vi "InertialControl.vi"() -> ()   [LabVIEW 2019]
doc: "high-level user control for inertial control"
uses:
  D:/Victor Sun/optical trap control/Kinesis/Thorlabs.MotionControl.Controls.dll
  Kinesis/Thorlabs.MotionControl.Controls.dll
  D:/Victor Sun/optical trap control/Kinesis/Thorlabs.MotionControl.KCube.InertialMotorCLI.dll
  Kinesis/Thorlabs.MotionControl.KCube.InertialMotorCLI.dll
panel:
  out "current state":string
  in  "stop data write loop":bool
  in  "start/stop write":bool
  in  "init file":bool
  in  "Folder path save":path
  in  "filename save":string="D:\\Victor Sun\\optical trap control\\output_test\\testposition"
  in  "decrease/reverse":bool
  in  "JogStepRev in":i32=250
  in  "JogStepFwd out":i32=500
  in  "position":i32
  in  "move to?":bool
  in  "increase/forward":bool
  out "JogStepRev out":i32
  out "JogStepFwd out":i32
  out "JogRate":i32
  out "JogAcceleration":i32
  out "JogMode":i32(ring)=1 items=["Continuous"=1, "Step"=2]
  out "StepRate":i32
  out "StepAcceleration":i32
  out "MaxVoltage":i32
  in  "stop motors":bool
  out "GetPosition":i32
  in  "Stop Button":bool
  in  "SerialNumber 2":string="97000019"
  in  "KCubeInertialMotorControl":refnum<k24>(container)
  # "Low-level parameters (which one of these to include)"
  # "Relative Position Control"
  # "Data Acquisition Settings"
  # "Absolute Position Control"
  # "Goto"
  # "Jog"
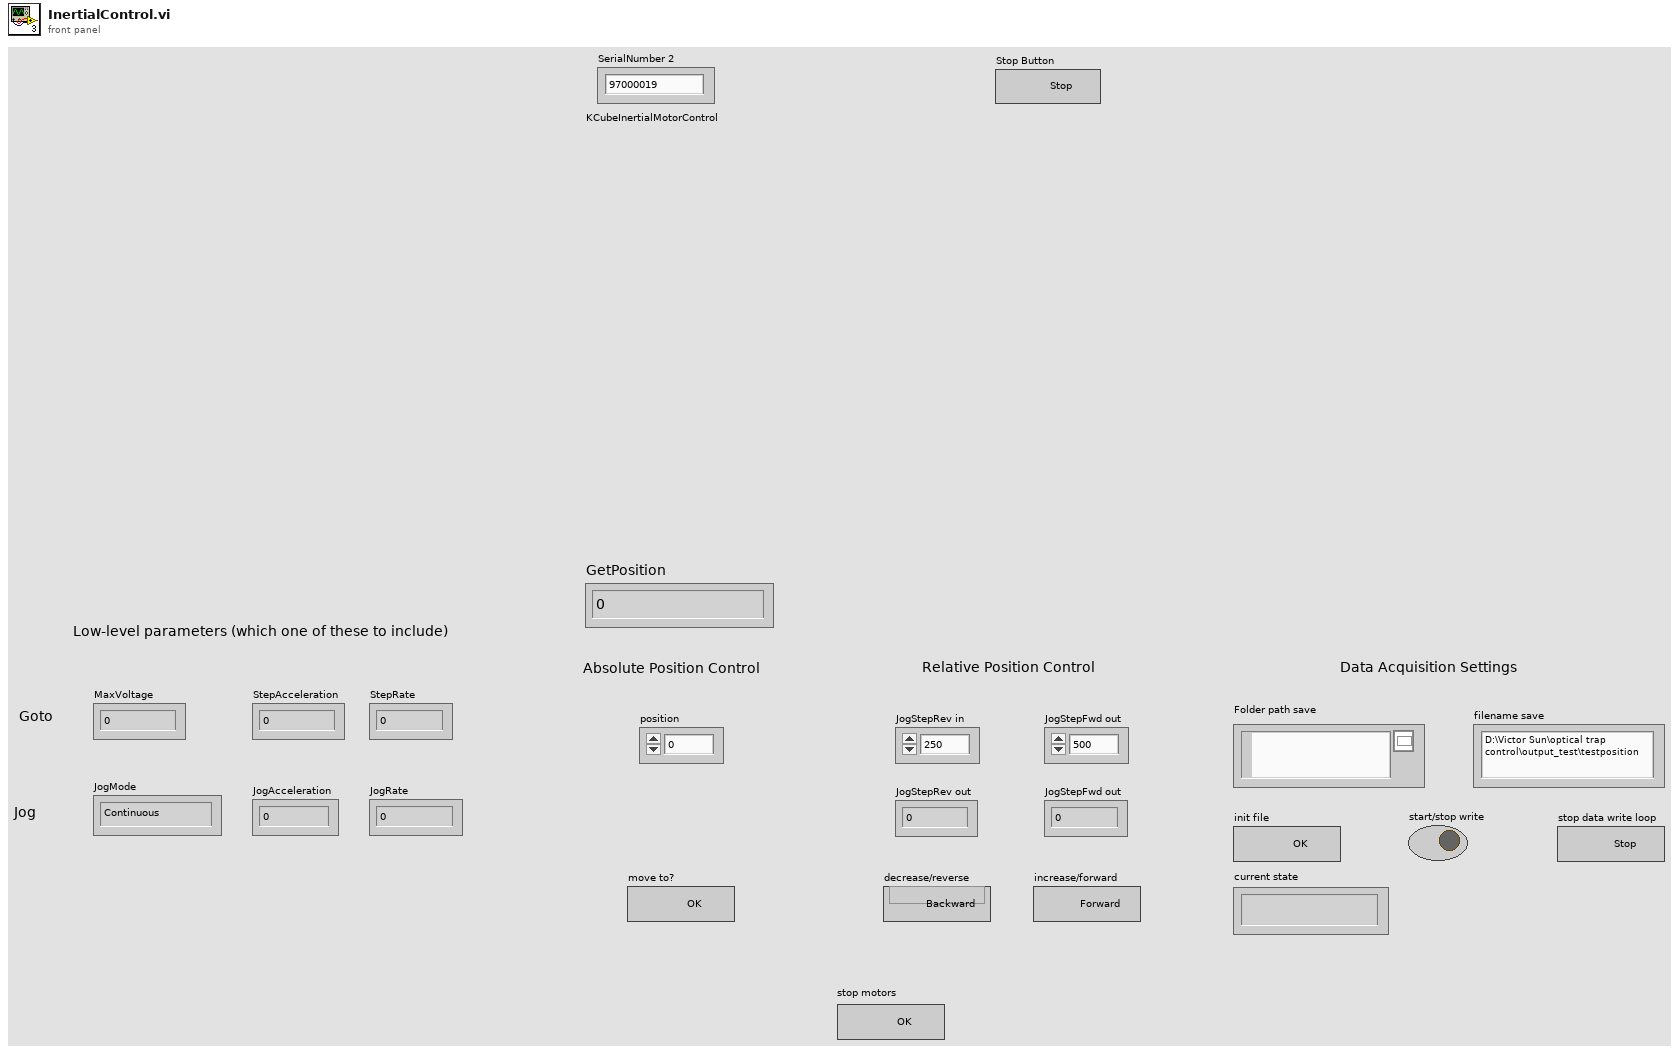
[diagram p1: front panel]
types:
  T1 = enum16{"waiting for init", "init", "waiting for write", "write", "stop"}
  T2 = cluster{"StepRate":i32, "StepAcceleration":i32, "MaxVoltage":i32}
  T3 = enum16{"waiting for init", "init", "waiting for write", "write", "stop", ""}
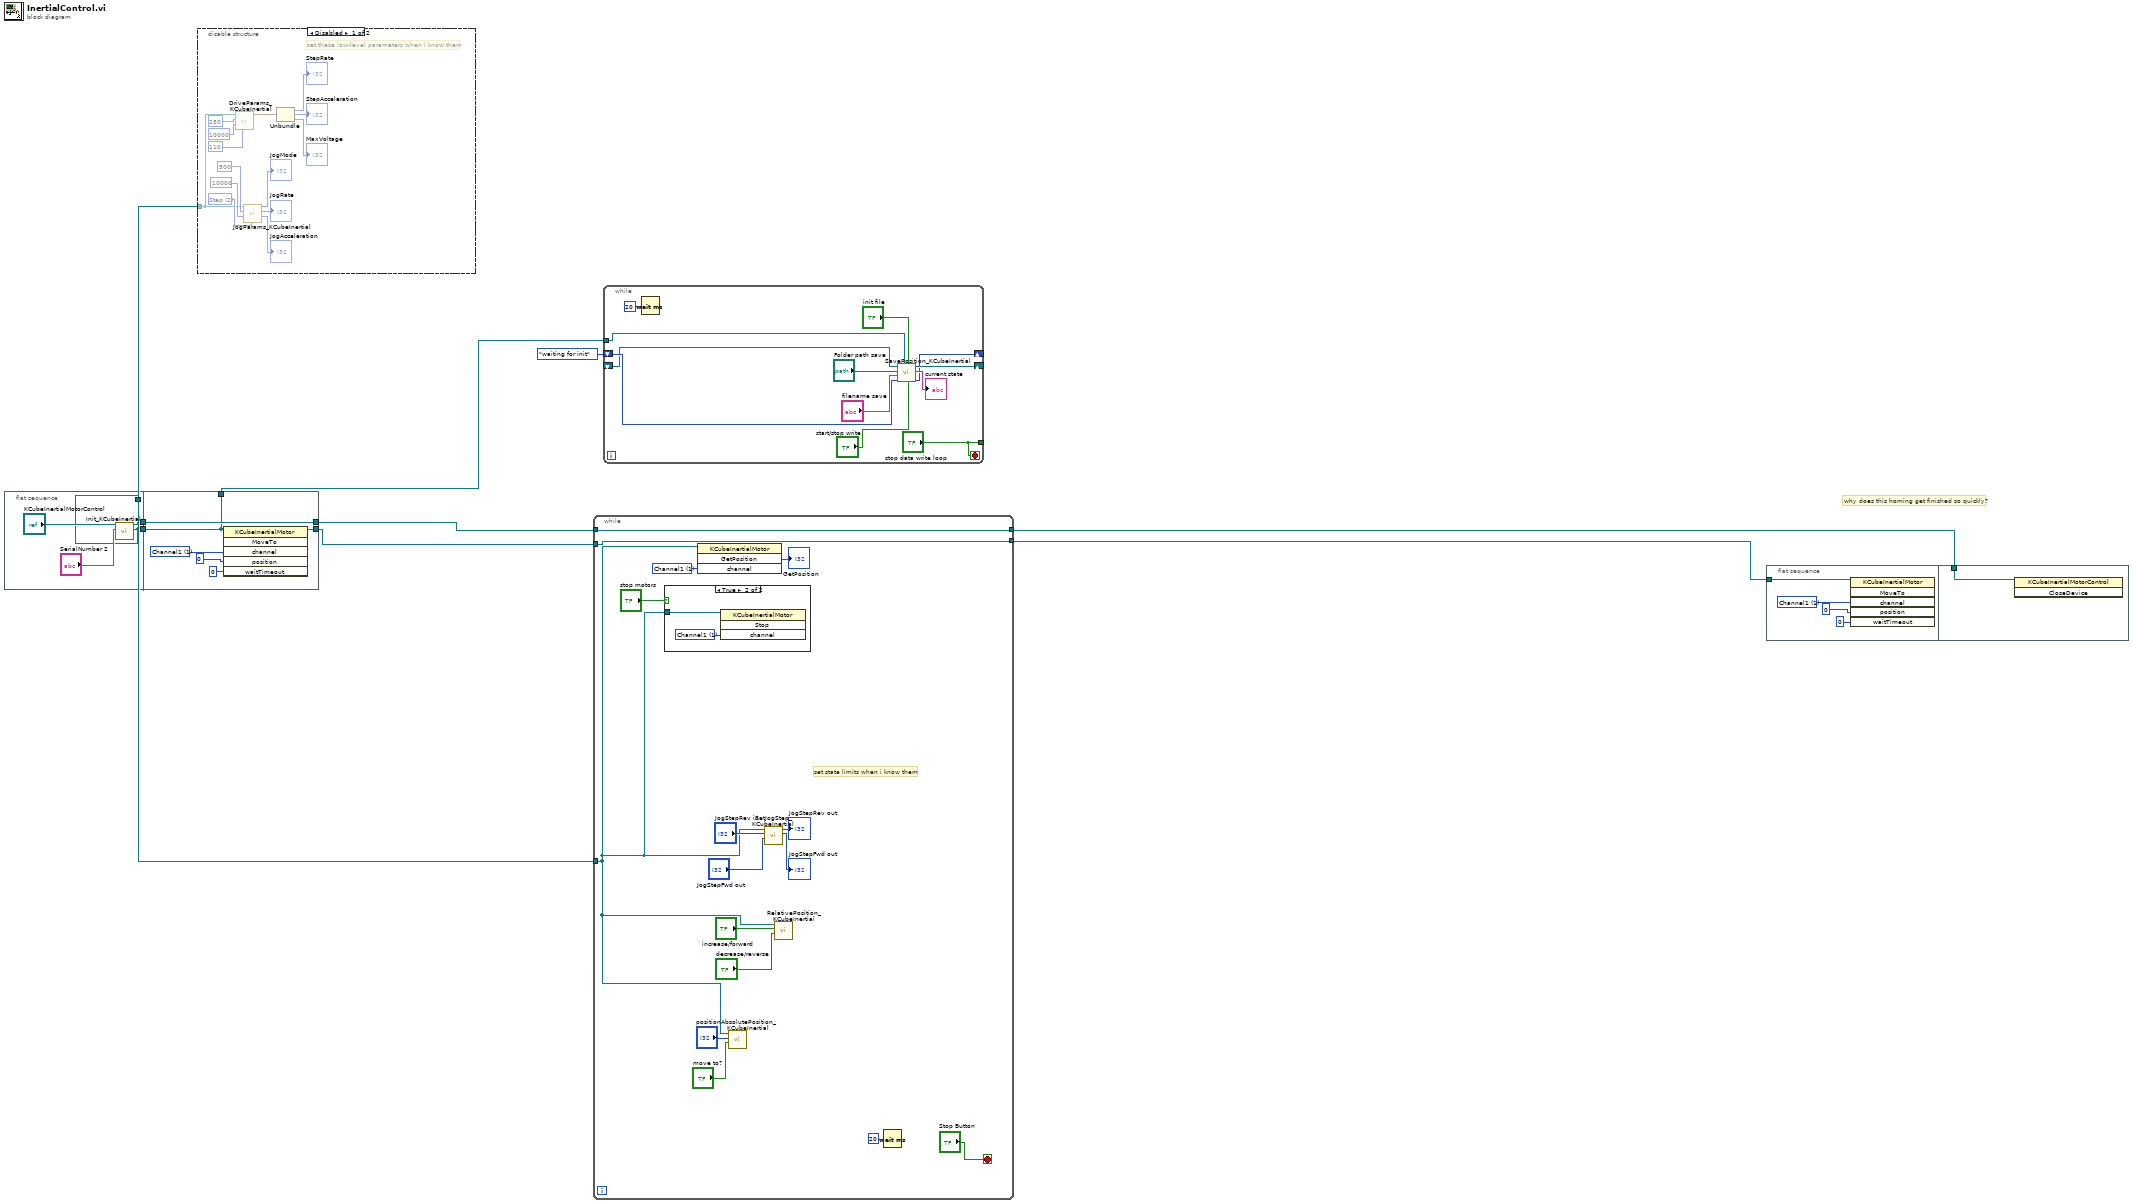
[diagram p0: block diagram]
diagram:
  # "why does this homing get finished so quickly?"
  n1 = flat-sequence {
    tunnel: [w10] -> w8
    tunnel: [w12] -> w6
    tunnel: [w10] -> w5
    tunnel: [w19] -> w9
    tunnel: w6 -> [w19]
    tunnel: w5 -> [w14]
    tunnel: [w15] -> w4
    tunnel: [w14] -> w1
    frame #0 {
      n2 = call "Init_KCubeInertial.vi"("SerialNumber in"="SerialNumber 2", ".NET Refnum in"="KCubeInertialMotorControl") -> ("Device"=w10:refnum<k24>, ".NET Refnum out"=w12:refnum<k24>)  [unwired: 7 in, 1 out]
    }
    frame #1 {
      w18 = 1 items=["Channel1"=1, "Channel2"=2, "Channel3"=3, "Channel4"=4] ("channel")
      n3 = invoke class="KCubeInertialMotor" method="MoveTo"(reference=w14, "channel"=w18, "position"=0, "waitTimeout"=0) -> (reference out=w15:refnum<k24>)  [unwired: 2 in, 5 out]
    }
  }
  n4 = disable-structure shown="Disabled" {
    disable-tunnel: w8 -> [w20 _]
    frame Disabled {
      w23 = 2 items=["Continuous"=1, "Step"=2] ("JogMode")
      # "set these low-level parameters when i know them"
      n5 = call "DriveParams_KCubeInertial.vi"("MaxVoltage"=110, "StepAcceleration"=10000, "StepRate"=250, ".NET Refnum in"=w20) -> ("Cluster"=w30:T2)  [unwired: 7 in]
      n6 = call "JogParams_KCubeInertial.vi"("JogMode in"=w23, "JogAcceleration in"=10000 ("JogAcceleration"), "JogRate in"=500 ("JogRate"), ".NET Refnum in"=w20) -> ("JogAcceleration out"=→"JogAcceleration":i32, "JogRate out"=→"JogRate":i32, "JogMode out"=→"JogMode":i32)  [unwired: 5 in]
      n7 = Unbundle(w30) -> ("StepRate"=→"StepRate":i32, "StepAcceleration"=→"StepAcceleration":i32, "MaxVoltage"=→"MaxVoltage":i32)
    }
    frame Enabled {
    }
  }
  n8 = while {
    tunnel: w9 -> [w48]
    tunnel: [w48] -> w7
    tunnel: w8 -> [w35]
    tunnel: w4 -> [w34]
    tunnel: [w34] -> w3
    stop <- "Stop Button" stop-if-true
    w46 = 1 items=["Channel1"=1, "Channel2"=2, "Channel3"=3, "Channel4"=4] ("channel")
    # "set state limits when i know them"
    n9 = case shown="True" "stop motors" {
      tunnel: w35 -> [_ w50]
      frame False {
      }
      frame True {
        w51 = 1 items=["Channel1"=1, "Channel2"=2, "Channel3"=3, "Channel4"=4] ("channel")
        n10 = invoke class="KCubeInertialMotor" method="Stop"(reference=w50, "channel"=w51) -> ()  [unwired: 2 in, 4 out]
      }
    }
    n11 = invoke class="KCubeInertialMotor" method="GetPosition"(reference=w35, "channel"=w46) -> ("GetPosition"=→"GetPosition":i32)  [unwired: 2 in, 3 out]
    n12 = call "AbsolutePosition_KCubeInertial.vi"("go to?"="move to?", "set absolute position"="position", ".NET Refnum in"=w35) -> ()  [unwired: 9 in]
    n13 = call "SetJogStep_KCubeInertial.vi"("JogStepFwd in"="JogStepFwd out", "JogStepRev in"="JogStepRev in", ".NET Refnum in"=w35) -> ("JogStepFwd out"=→"JogStepFwd out":i32, "JogStepRev out"=→"JogStepRev out":i32)  [unwired: 7 in]
    n14 = call "RelativePosition_KCubeInertial.vi"("decrease/reverse"="decrease/reverse", "increase/forward"="increase/forward", ".NET Refnum in"=w35) -> ()  [unwired: 9 in]
    n15 = Wait (ms)(milliseconds to wait=u32 20) -> ()  [unwired: 1 out]
  }
  n16 = while {
    shift-right: [w56] -> _
    shift-left: T1."waiting for init" -> [w55]
    tunnel: w1 -> [w53]
    shift-right: [w62] -> _
    shift-left: _ -> [w52]
    tunnel: ["stop data write loop"] -> _
    stop <- "stop data write loop" stop-if-true
    n17 = Wait (ms)(milliseconds to wait=u32 20) -> ()  [unwired: 1 out]
    n18 = call "SavePosition_KCubeInertial.vi"("start/stop write"="start/stop write", "init file"="init file", "Device"=w53, "state in"=w55, "filename save"="filename save", "Folder path save"="Folder path save", "Byte Stream File in"=w52) -> ("state out"=w56:T3, "current state"=→"current state":string, "Byte Stream File out"=w62:refnum<file>)  [unwired: 2 in]
  }
  n19 = flat-sequence {
    tunnel: w3 -> [w64]
    tunnel: w7 -> [w68]
    frame #0 {
      w67 = 1 items=["Channel1"=1, "Channel2"=2, "Channel3"=3, "Channel4"=4] ("channel")
      n20 = invoke class="KCubeInertialMotor" method="MoveTo"(reference=w64, "channel"=w67, "position"=0, "waitTimeout"=0) -> ()  [unwired: 2 in, 6 out]
    }
    frame #1 {
      n21 = invoke class="KCubeInertialMotorControl" method="CloseDevice"(reference=w68) -> ()  [unwired: 2 in, 3 out]
    }
  }
